vi "Parse Array.vi"(8 "error in (no error)":errorcluster, 10 "Index In":i32, 11 "JSON String":string) -> (0 "error out":errorcluster, 2 "Index Out":i32, 3 "JSON Value out":refnum<class "JSON Value.lvclass">)   [LabVIEW 2016, in "JSON Value.lvclass"]
uses:
  JSON Value.lvclass
  subVIs/Errors.ctl
  New JSON Value/New JSON (Value[]).vi
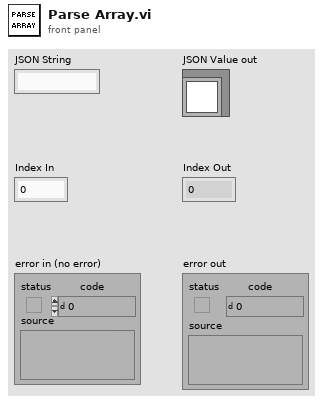
[diagram p1: front panel]
types:
  T1 = typedef "JSON Value.lvclass/Errors.ctl" = enum8{"No key", "Key path type", "Array OOB", "Type Mismatch", "Invalid Token"}
  T2 = typedef "JSON Value.lvclass/Token Type.ctl" = enum8{"NONE", "CURLY_OPEN", "CURLY_CLOSE", "SQUARED_OPEN", "SQUARED_CLOSE", "COLON", "COMMA", "STRING", "NUMBER", "TRUE", "FALSE", "NULL"}
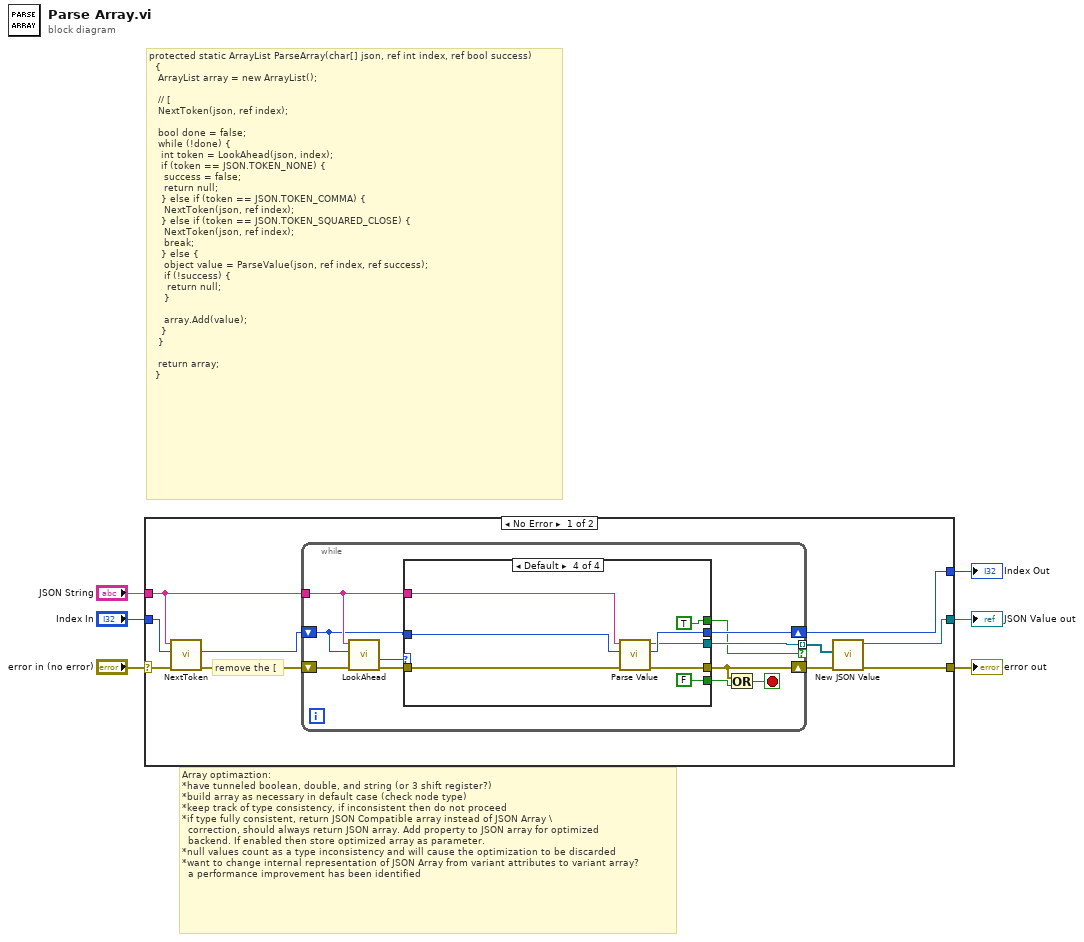
[diagram p0: block diagram]
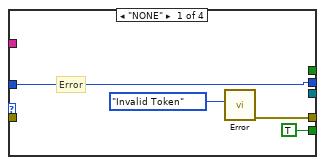
[diagram p2: hidden frame]
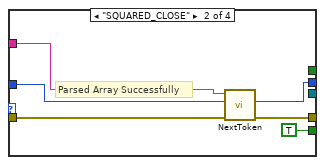
[diagram p3: hidden frame]
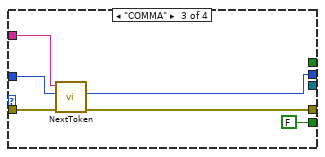
[diagram p4: hidden frame]
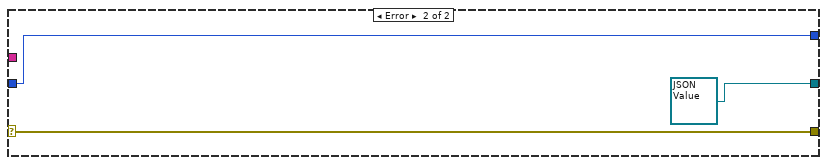
[diagram p5: hidden frame]
diagram:
  # "Array optimaztion:\n*have tunneled boolean, double, and string (or 3 shift register?)\n*build array as necessary in default case (check node type)\n*keep track of type consistency, if inconsistent then do not proceed\n*if type fully consistent, return JSON Compatible array instead of JSON Array \\\n  correction, should always return JSON array. Add property to JSON array for optimized\n  backend. If enabled then store optimized array as parameter.\n*null values count as a type inconsistency and will cause the optimization to be discarded\n*want to change internal representation of JSON Array from variant attributes to variant array?\n  a performance improvement has been identified"
  # "protected static ArrayList ParseArray(char[] json, ref int index, ref bool success)\n\t\t{\n\t\t\tArrayList array = new ArrayList();\n\n\t\t\t// [\n\t\t\tNextToken(json, ref index);\n\n\t\t\tbool done = false;\n\t\t\twhile (!done) {\n\t\t\t\tint token = LookAhead(json, index);\n\t\t\t\tif (token == JSON.TOKEN_NONE) {\n\t\t\t\t\tsuccess = false;\n\t\t\t\t\treturn null;\n\t\t\t\t} else if (token == JSON.TOKEN_COMMA) {\n\t\t\t\t\tNextToken(json, ref index);\n\t\t\t\t} else if (token == JSON.TOKEN_SQUARED_CLOSE) {\n\t\t\t\t\tNextToken(json, ref index);\n\t\t\t\t\tbreak;\n\t\t\t\t} else {\n\t\t\t\t\tobject value = ParseValue(json, ref index, ref success);\n\t\t\t\t\tif (!success) {\n\t\t\t\t\t\treturn null;\n\t\t\t\t\t}\n\n\t\t\t\t\tarray.Add(value);\n\t\t\t\t}\n\t\t\t}\n\n\t\t\treturn array;\n\t\t}"
  n1 = case shown="No Error" "error in (no error)" {
    selector: "error in (no error)" -> [w16 w53]
    tunnel: [w8 w53] -> w5
    tunnel: "Index In" -> [w15 w54]
    tunnel: [w12 w54] -> w3
    tunnel: [w11 refnum<class "JSON Value.lvclass"> refnum ("JSON out")] -> w1
    tunnel: "JSON String" -> [w7 _]
    frame No Error {
      # "remove the ["
      n2 = call "NextToken.vi"("error in (no error)"=w16, "Index In"=w15, "JSON String"=w7) -> ("error out"=w13:errorcluster, "Index Out"=w14:i32)  [unwired: 6 in, 1 out]
      n3 = while {
        shift-right: [w24] -> w12
        shift-left: w14 -> [w17]
        tunnel: w7 -> [w18]
        shift-right: [w21] -> w9
        shift-left: w13 -> [w27]
        tunnel: [w20] -> w10 mode=indexing if=w19
        stop <- w22 stop-if-true
        n4 = call "LookAhead.vi"("error in (no error)"=w27, "Index"=w17, "JSON String"=w18) -> ("error out"=w25:errorcluster, "TOKEN"=w26:T2)  [unwired: 7 in]
        n5 = case shown="Default" w26 {
          tunnel: w25 -> [_ w37 w41 w51]
          tunnel: [TRUE TRUE FALSE FALSE] -> w23
          tunnel: w17 -> [w30 w36 w42 w50]
          tunnel: w18 -> [_ w35 w43 w49]
          tunnel: [w30 w33 w39 w48] -> w24
          tunnel: [w29 w34 w40 w46] -> w21
          tunnel: [_ _ _ w45] -> w20
          tunnel: [_ _ _ TRUE] -> w19
          frame "NONE" {
            # "Error"
            n6 = call "Error.vi"("Error"=Errors."Invalid Token") -> ("error out"=w29:errorcluster)  [unwired: 9 in]
          }
          frame "SQUARED_CLOSE" {
            # "Parsed Array Successfully"
            n7 = call "NextToken.vi"("error in (no error)"=w37, "Index In"=w36, "JSON String"=w35) -> ("error out"=w34:errorcluster, "Index Out"=w33:i32)  [unwired: 6 in, 1 out]
          }
          frame "COMMA" {
            n8 = call "NextToken.vi"("error in (no error)"=w41, "Index In"=w42, "JSON String"=w43) -> ("error out"=w40:errorcluster, "Index Out"=w39:i32)  [unwired: 6 in, 1 out]
          }
          frame Default {
            n9 = call "Parse Value.vi"("error in (no error)"=w51, "Index In"=w50, "JSON String"=w49) -> ("error out"=w46:errorcluster, "Index Out"=w48:i32, "JSON Value out"=w45:refnum<class "JSON Value.lvclass">)  [unwired: 6 in]
          }
        }
        n10 = Or(x=w21, y=w23) -> (x .or. y?=w22:bool)
      }
      n11 = call-poly "New JSON Value.vi"("error in (no error)"=w9, "JSON Datatypes"=w10) -> ("error out"=w8:errorcluster, "JSON Value out"=w11:refnum<class "JSON Value.lvclass">)  [unwired: 8 in]
    }
    frame Error {
    }
  }
  "error out" <- w5
  "Index Out" <- w3
  "JSON Value out" <- w1
